vi "release_port.vi"() -> ()   [LabVIEW 2009]
panel:
  out "error out":errorcluster
  in  "VISA resource name":refnum<visa-resource-name>
  # "Port Release"
  # "If there is an error connecting to an instrument, there is a good chance that there is an old VISA session still open.  Use this VI to make sure that there are no remaining VISA sessions over any of the ports.  Select the offending port in \"VISA resource name\" and click run to close any remaining sessions.  There should be no errors in the \"error out\" display."
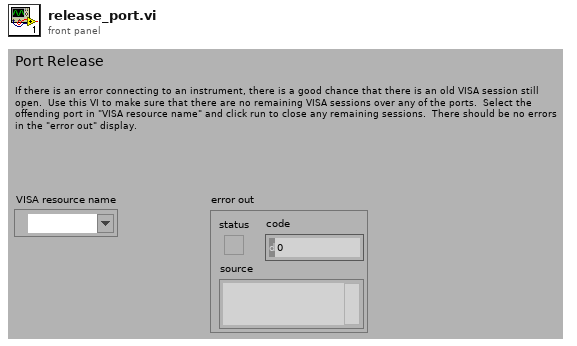
[diagram p1: front panel]
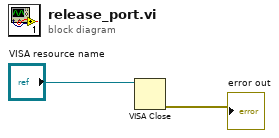
[diagram p0: block diagram]
diagram:
  n1 = VISA Close(VISA resource name="VISA resource name") -> (error out=→"error out":errorcluster)  [unwired: 1 in]
